vi "TP Buffer Add New Data Packet to Connection.vi"(0 "Connection Cluster":T3, 5 "CAN frame":T1 {"payload" format="%x"; "timestamp" format="%<%.7X\n%x>T"; "type" items=["CAN Data"=0, "CAN Remote"=1, "CAN Bus Error"=2, "J1939 Data"=192, "Delay"=224, "Log Trigger"=225, "Start Trigger"=226]; "identifier" format="%x"}, 11 "error in (no error)":errorcluster) -> (4 "Connection Cluster Out":T3, 6 "Frame Mismatch?":bool, 8 "Message Complete?":bool, 15 "error out":errorcluster)   [LabVIEW 2013, in "J1939.lvlib"]
uses:
  J1939.lvlib
  TP Buffer Connection Cluster.ctl
  <vilib>/xnet/xnet.llb/XNET Frame CAN.ctl
  <vilib>/xnet/xnet.llb/XNET Frame Type CAN.ctl
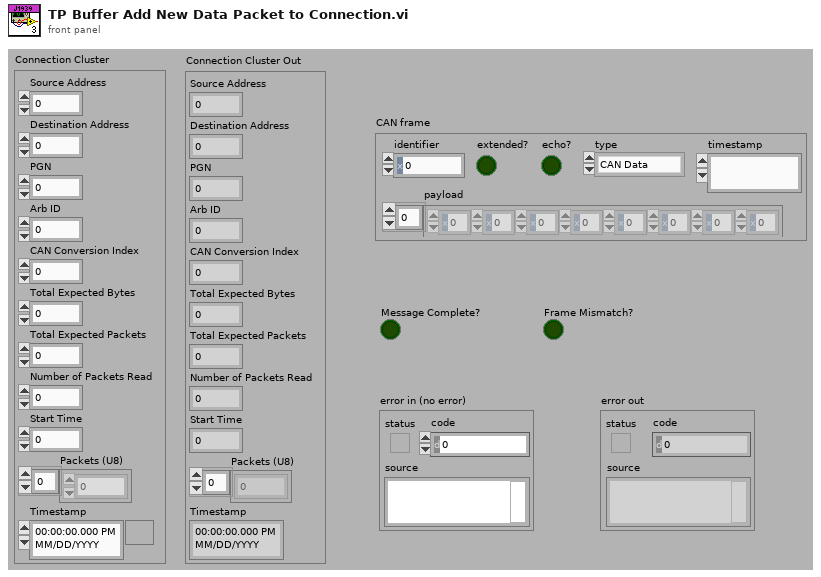
[diagram p1: front panel]
types:
  T1 = typedef "XNET Frame CAN.ctl" = cluster{"timestamp":timestamp, "payload":u8[], "identifier":u32, "type":T2, "extended?":bool, "echo?":bool}
  T2 = typedef "XNET Frame Type CAN.ctl" = u8
  T3 = typedef "J1939.lvlib/TP Buffer Connection Cluster.ctl" = cluster{"Source Address":u8, "Destination Address":u8, "PGN":u32, "Arb ID":u32, "CAN Conversion Index":u32, "Total Expected Bytes":u16, "Total Expected Packets":u8, "Number of Packets Read":u8, "Start Time":u32, "Packets (U8)":u8[], "Timestamp":timestamp}
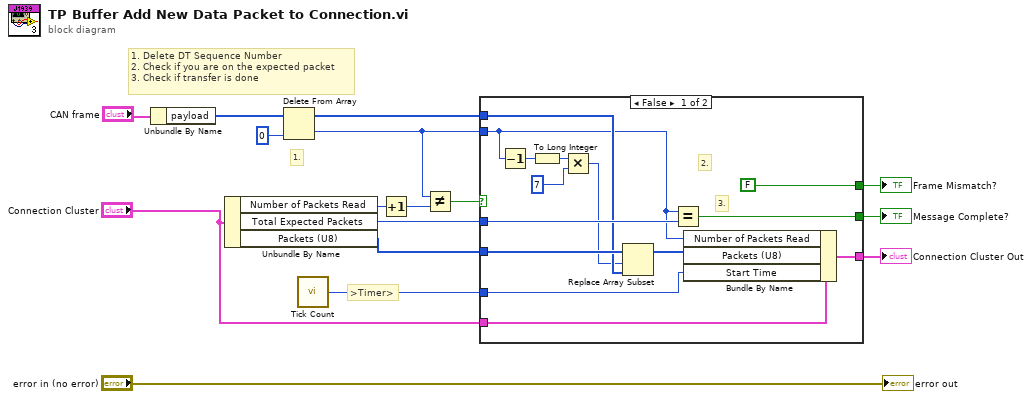
[diagram p0: block diagram]
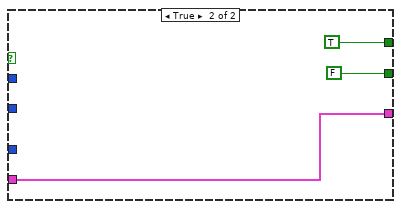
[diagram p2: hidden frame]
diagram:
  # "1."
  # "1. Delete DT Sequence Number\n2. Check if you are on the expected packet\n3. Check if transfer is done"
  # ">Timer>"
  n1 = Unbundle By Name("CAN frame") -> ("payload"=w13:u8[])
  n2 = Unbundle By Name("Connection Cluster") -> ("Number of Packets Read"=w6:u8, "Total Expected Packets"=w12:u8, "Packets (U8)"=w11:u8[])
  n3 = Delete From Array(array=w13, index=0) -> (deleted portion=w4:u8, array with subset deleted=w9:u8[])  [unwired: 1 in]
  n4 = call "Tick Count"() -> ("Tick Count(mSec)"=w16:u32)
  n5 = Increment(x=w6) -> (x+1=w5:u8)
  n6 = Not Equal?(x=w4, y=w5) -> (x != y?=w3:bool)
  n7 = case shown="False" w3 {
    tunnel: w16 -> [w30 _]
    tunnel: "Connection Cluster" -> [w29 w33]
    tunnel: w12 -> [w28 _]
    tunnel: w11 -> [w27 _]
    tunnel: w9 -> [w25 _]
    tunnel: [w23 w33] -> w8
    tunnel: [w20 FALSE] -> w7
    tunnel: w4 -> [w19 _]
    tunnel: [FALSE TRUE] -> w2
    frame False {
      # "3."
      # "2."
      n8 = Decrement(x=w19) -> (x-1=w22:u8)
      n9 = To Long Integer(number=w22) -> (32bit integer=w17:i32)
      n10 = Multiply(x=w17, y=7 ("x")) -> (x*y=w24:i32)
      n11 = Replace Array Subset(array=w27, new element=w25, index=w24) -> (w21:u8[])
      n12 = Equal?(x=w19, y=w28) -> (x = y?=w20:bool)
      n13 = Bundle By Name(cluster=w29, "Number of Packets Read"=w19, "Packets (U8)"=w21, "Start Time"=w30) -> (w23:T3)
    }
    frame True {
    }
  }
  "Connection Cluster Out" <- w8
  "Message Complete?" <- w7
  "Frame Mismatch?" <- w2
  "error out" <- "error in (no error)"
